vi "Escape JSON string.vi"(8 "error in (no error)":errorcluster, 11 "Text (unscaped)":string) -> (0 "error out":errorcluster, 3 "Text (escaped)":string)   [LabVIEW 2011, in "JSON Value.lvclass"]
uses:
  JSON Value/JSON Value.lvclass
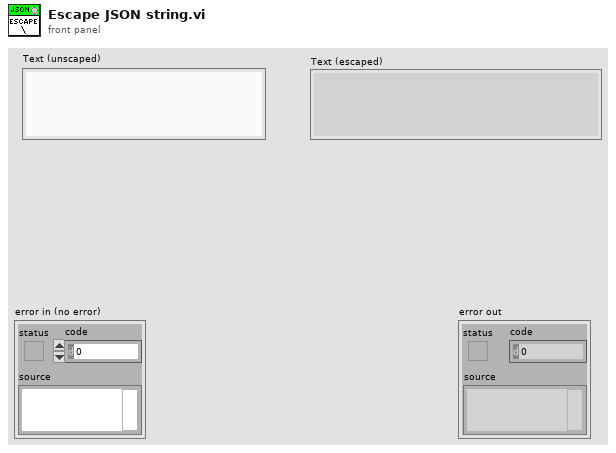
[diagram p1: front panel]
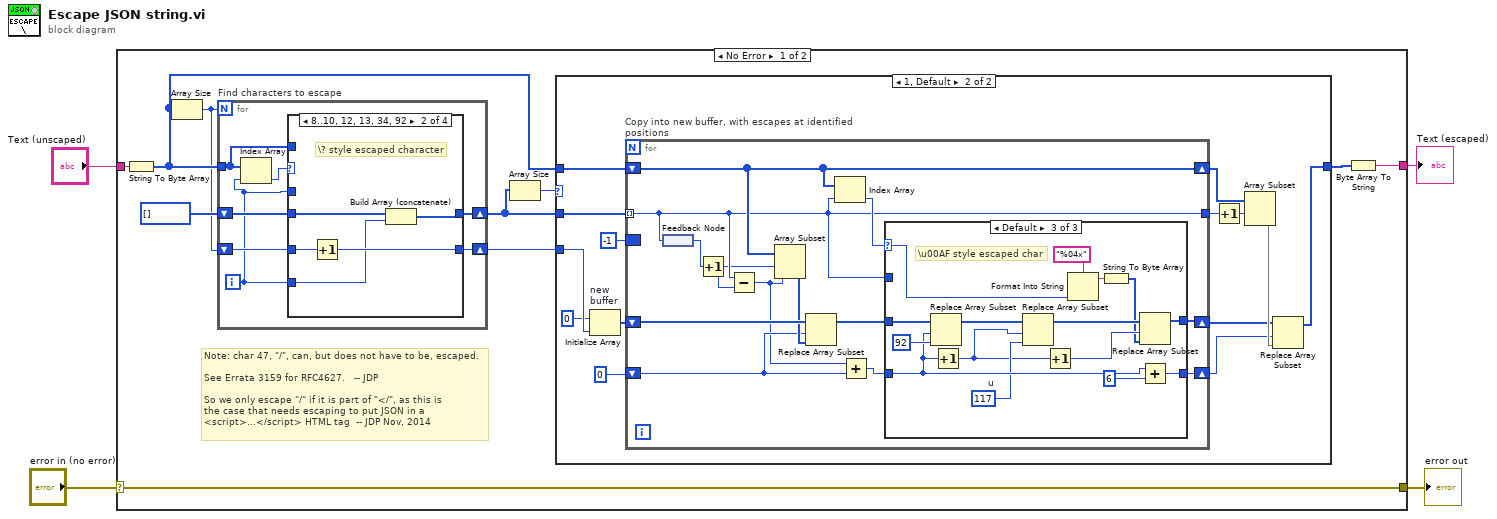
[diagram p0: block diagram]
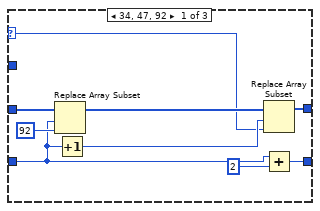
[diagram p3: hidden frame]
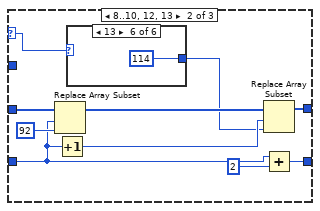
[diagram p4: hidden frame]
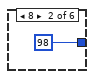
[diagram p6: hidden frame]
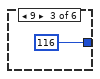
[diagram p7: hidden frame]
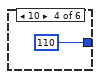
[diagram p8: hidden frame]
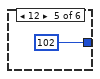
[diagram p9: hidden frame]
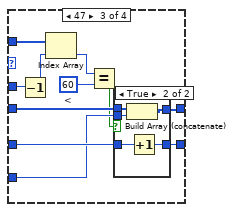
[diagram p11: hidden frame]
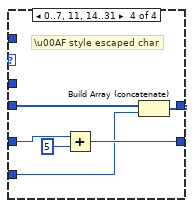
[diagram p13: hidden frame]
diagram:
  n1 = case shown="No Error" "error in (no error)" {
    selector: "error in (no error)" -> [w14 w121]
    tunnel: [w14 w121] -> w3
    tunnel: "Text (unscaped)" -> [w13 w120]
    tunnel: [w12 w120] -> w1
    frame No Error {
      # "Note: char 47, \"/\", can, but does not have to be, escaped.\n\nSee Errata 3159 for RFC4627.   -- JDP\n\nSo we only escape \"/\" if it is part of \"</\", as this is\nthe case that needs escaping to put JSON in a\n<script>...</script> HTML tag  -- JDP Nov, 2014"
      n2 = String To Byte Array(string=w13) -> (unsigned byte array=w6:u8[])
      n3 = Array Size(array=w6) -> (size(s)=w5:i32)
      n4 = for "Find characters to escape" {
        N: w5 -> [_]
        tunnel: w6 -> [w83]
        shift-right: [w87] -> w10
        shift-left: w5 -> [w88]
        shift-right: [w86] -> w8
        shift-left: i32[] [] -> [w85]
        i -> [w82]
        n5 = Index Array(array=w83, index=w82) -> (element=w84:u8)
        n6 = case shown="8..10, 12, 13, 34, 92" w84 {
          tunnel: w88 -> [w90 w95 w106 w116]
          tunnel: [w90 w94 w105 w119] -> w87
          tunnel: [w89 w93 w104 w118] -> w86
          tunnel: w85 -> [w89 w92 w103 w117]
          tunnel: w82 -> [_ w91 w102 w114]
          tunnel: w83 -> [_ _ w99 _]
          tunnel: w82 -> [_ _ w101 _]
          frame Default {
            # "Not escaped"
          }
          frame 8..10, 12, 13, 34, 92 {
            # "\\? style escaped character"
            n7 = Increment(x=w95) -> (x+1=w94:i32)
            n8 = Build Array (concatenate)(w92, w91) -> (w93:i32[])
          }
          frame 47 {
            w97 = u8 60  # <
            n9 = Decrement(x=w101) -> (x-1=w100:i32)
            n10 = Index Array(array=w99, index=w100) -> (element=w98:u8)
            n11 = Equal?(x=w98, y=w97) -> (x = y?=w96:bool)
            n12 = case shown="True" w96 {
              tunnel: w106 -> [w107 w113]
              tunnel: [w107 w112] -> w105
              tunnel: [w108 w111] -> w104
              tunnel: w103 -> [w108 w110]
              tunnel: w102 -> [_ w109]
              frame False {
              }
              frame True {
                n13 = Build Array (concatenate)(w110, w109) -> (w111:i32[])
                n14 = Increment(x=w113) -> (x+1=w112:i32)
              }
            }
          }
          frame 0..7, 11, 14..31 {
            # "\\u00AF style escaped char"
            n15 = Add(x=w116, y=5) -> (x+y=w119:i32)
            n16 = Build Array (concatenate)(w117, w114) -> (w118:i32[])
          }
        }
      }
      n17 = Array Size(array=w8) -> (size(s)=w7:i32)
      n18 = case shown="1, Default" w7 {
        tunnel: w10 -> [_ w29]
        tunnel: w8 -> [_ w27]
        tunnel: w6 -> [w15 w26]
        tunnel: [w15 w17] -> w9
        frame 0 {
          # "Nothing to escape"
        }
        frame 1, Default {
          n19 = Initialize Array "new\nbuffer"(u8 0, w29) -> (w25:u8[])
          n20 = for "Copy into new buffer, with escapes at identified positions" {
            tunnel: w27 -> [w32] mode=indexing
            shift-right: [w36] -> w20
            shift-left: w26 -> [w36]
            border: -1 -> [_]
            shift-right: [w35] -> w18
            shift-left: 0 ("x+1") -> [w34]
            shift-right: [w37] -> w21
            shift-left: w25 -> [w40]
            tunnel: [w32] -> w19
            n21 = feedback-in #1(w32) -> ()
            n22 = feedback #1() -> (w41:i32)
            n23 = Increment(x=w41) -> (x+1=w31:i32)
            n24 = Subtract(x=w32, y=w31) -> (x-y=w30:i32)
            n25 = Array Subset(array=w36, index=w31, length=w30) -> (w39:u8[])
            n26 = Replace Array Subset(array=w40, new element=w39, index=w34) -> (w38:u8[])
            n27 = Index Array(array=w36, index=w32) -> (element=w42:u8)
            n28 = Add(x=w30, y=w34) -> (x+y=w33:i32)
            n29 = case shown="Default" w42 {
              selector: w42 -> [w47 w53 w73]
              tunnel: w38 -> [w51 w61 w81]
              tunnel: w32 -> [_ _ _]
              tunnel: [w46 w57 w79] -> w37
              tunnel: w33 -> [w43 w54 w76]
              tunnel: [w44 w55 w77] -> w35
              frame 34, 47, 92 {
                n30 = Replace Array Subset(array=w51, new element=u8 92 ("new element/subarray"), index=w43) -> (w49:u8[])
                n31 = Increment(x=w43) -> (x+1=w48:i32)
                n32 = Replace Array Subset(array=w49, new element=w47, index=w48) -> (w46:u8[])
                n33 = Add(x=w43, y=2) -> (x+y=w44:i32)
              }
              frame 8..10, 12, 13 {
                n34 = Replace Array Subset(array=w61, new element=u8 92 ("new element/subarray"), index=w54) -> (w59:u8[])
                n35 = Increment(x=w54) -> (x+1=w58:i32)
                n36 = case shown="13" w53 {
                  tunnel: [_ u8 98 u8 116 u8 110 u8 102 u8 114] -> w52
                  frame 0, Default {
                  }
                  frame 8 {
                  }
                  frame 9 {
                  }
                  frame 10 {
                  }
                  frame 12 {
                  }
                  frame 13 {
                  }
                }
                n37 = Replace Array Subset(array=w59, new element=w52, index=w58) -> (w57:u8[])
                n38 = Add(x=w54, y=2) -> (x+y=w55:i32)
              }
              frame Default {
                w72 = u8 117  # u
                # "\\u00AF style escaped char"
                n39 = Replace Array Subset(array=w81, new element=u8 92 ("new element/subarray"), index=w76) -> (w71:u8[])
                n40 = Increment(x=w76) -> (x+1=w69:i32)
                n41 = Replace Array Subset(array=w71, new element=w72, index=w69) -> (w70:u8[])
                n42 = Increment(x=w69) -> (x+1=w68:i32)
                n43 = Format Into String(format string="%04x", w73) -> (resulting string=w74:string)  [unwired: 2 in, 1 out]
                n44 = String To Byte Array(string=w74) -> (unsigned byte array=w67:u8[])
                n45 = Replace Array Subset(array=w70, new element=w67, index=w68) -> (w79:u8[])
                n46 = Add(x=w76, y=6) -> (x+y=w77:i32)
              }
            }
          }
          n47 = Increment(x=w19) -> (x+1=w16:i32)
          n48 = Array Subset(array=w20, index=w16) -> (w22:u8[])  [unwired: 1 in]
          n49 = Replace Array Subset(array=w21, new element=w22, index=w18) -> (w17:u8[])
        }
      }
      n50 = Byte Array To String(unsigned byte array=w9) -> (string=w12:string)
    }
    frame Error {
    }
  }
  "error out" <- w3
  "Text (escaped)" <- w1
